vi "Check All Hardware Status.vi"(8 "error in (no error)":errorcluster caption="entrée d'erreur (pas d'erreur)", 11 "Control en entrée":refnum<class "Control-Server.lvclass">) -> (0 "error out":errorcluster caption="sortie d'erreur", 2 "HARDWARE":bool, 3 "Control en sortie":refnum<class "Control-Server.lvclass">)   [LabVIEW 2015, in "Control-Server.lvclass"]
uses:
  Control-Server.lvclass
  dependecies/ControlsVIs/Clusters-def/Message types.ctl
  dependecies/ControlsVIs/Clusters-def/Standard Command.ctl
  dependecies/ControlsVIs/Clusters-def/SERVER-Commands.ctl
  dependecies/ControlsVIs/Clusters-def/CONTROL-Reply-Allconnect.ctl
  Control-Server.lvclass/Control-Server.ctl
  GeneralFunctionality/GeneralFunctionality.lvclass/GeneralFunctionality.ctl
  Delay Line/DelayLine.lvclass
  Detector/Detector.lvclass
  Oscilloscope/Oscilloscope.lvclass
  DAQmxTasks/DAQmxTaskContainer/DAQmxTaskContainer.lvclass
  Message/Message.lvclass
  GeneralFunctionality/GeneralFunctionality.lvclass
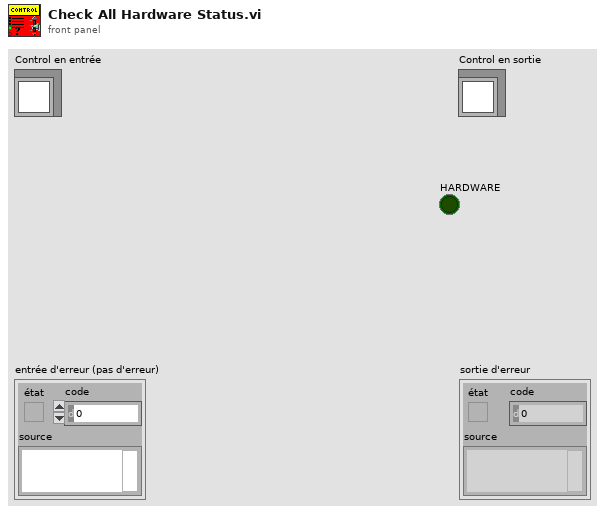
[diagram p1: front panel]
types:
  T1 = typedef "Control-Server.lvclass/CONTROL-Reply-Allconnect.ctl" = cluster{"On/Off":bool, "error":errorcluster}
  T2 = typedef "Control-Server.lvclass/SERVER-Commands.ctl" = string
  T3 = typedef "Standard Command.ctl" = cluster{"command":string, "data":variant}
  T4 = typedef "Message types.ctl" = string
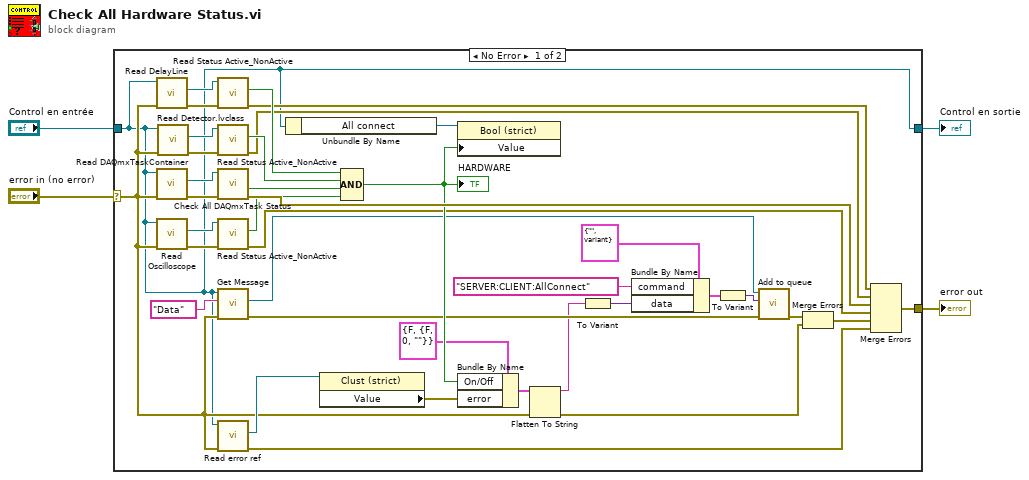
[diagram p0: block diagram]
diagram:
  n1 = case shown="No Error" "error in (no error)" {
    selector: "error in (no error)" -> [w13 w44]
    tunnel: [w30 w44] -> w3
    tunnel: [w6 w43] -> w1
    tunnel: "Control en entrée" -> [w6 w43]
    frame No Error {
      n2 = call "Read DelayLine.vi"("error in (no error)"=w13, "Control in"=w6) -> ("error out"=w40:errorcluster, "DelayLine.lvclass"=w39:refnum<class "DelayLine.lvclass">)  [unwired: 7 in, 1 out]
      n3 = call-dynamic "Read DAQmxTaskContainer.vi"("error in (no error)"=w13, "Control in"=w6) -> ("error out"=w38:errorcluster, "DAQmxTaskContainer.lvclass"=w37:refnum<class "DAQmxTaskContainer.lvclass">)  [unwired: 7 in, 1 out]
      n4 = call "Read Oscilloscope.vi"("error in (no error)"=w13, "Control-Server en entrée"=w6) -> ("error out"=w12:errorcluster, "Oscilloscope.lvclass"=w11:refnum<class "Oscilloscope.lvclass">)  [unwired: 7 in, 1 out]
      n5 = call "Read Detector.lvclass.vi"("error in (no error)"=w13, "Control in"=w6) -> ("error out"=w42:errorcluster, "Detector.lvclass"=w41:refnum<class "Detector.lvclass">)  [unwired: 7 in, 1 out]
      n6 = call "Read Status Active_NonActive.vi"("error in (no error)"=w40, "GeneralFunctionality in"=w39) -> ("error out"=w33:errorcluster, "Status Active/NonActive"=w36:bool)  [unwired: 7 in, 1 out]
      n7 = call "Read Status Active_NonActive.vi"("error in (no error)"=w42, "GeneralFunctionality in"=w41) -> ("error out"=w32:errorcluster, "Status Active/NonActive"=w35:bool)  [unwired: 7 in, 1 out]
      n8 = call "Check All DAQmxTask Status.vi"("error in (no error)"=w38, "DAQmxTaskContainer en entrée"=w37) -> ("error out"=w31:errorcluster, "One at least active"=w34:bool)  [unwired: 6 in, 2 out]
      n9 = call "Read Status Active_NonActive.vi"("error in (no error)"=w12, "GeneralFunctionality in"=w11) -> ("error out"=w9:errorcluster, "Status Active/NonActive"=w10:bool)  [unwired: 7 in, 1 out]
      n10 = call "Get Message.vi"("error in (no error)"=w13, "Message type"=T4 "Data", "GeneralFunctionality en entrée"=w6) -> ("error out"=w28:errorcluster, "Message.lvclass"=w26:refnum<class "Message.lvclass">)  [unwired: 6 in, 1 out]
      n11 = call "Read error ref.vi"("error in (no error)"=w13, "GeneralFunctionality in"=w6) -> ("error out"=w7:errorcluster, "error"=w17:refnum<vi>)  [unwired: 7 in, 1 out]
      n12 = Unbundle By Name(w6) -> ("All connect"=w5:refnum<vi>)
      n13 = property class="Clust (strict)"(reference=w17) -> ("Value"=w19:errorcluster)  [unwired: 1 in, 2 out]
      n14 = Compound Arithmetic op=AND ("Opérateur arithmétique")(w36, w35, w34, w10) -> (w29:bool)
      "HARDWARE" <- w29
      n15 = property class="Bool (strict)"(reference=w5, "Value"=w29) -> ()  [unwired: 1 in, 2 out]
      n16 = Bundle By Name(cluster=T1 {"On/Off"=FALSE, "error"={"status"=FALSE, "code"=0, "source"=""}} ("output cluster"), "On/Off"=w29, "error"=w19) -> (w16:T1)
      n17 = Flatten To String(anything=w16, error in (no error)=w13) -> (data string=w15:string, error out=w14:errorcluster)  [unwired: 2 in, 1 out]
      n18 = To Variant(anything=w15) -> (Variant=w22:variant)
      n19 = Bundle By Name(cluster=T3 {"command"="", "data"=variant} ("input cluster"), "command"=T2 "SERVER:CLIENT:AllConnect" ("Commands"), "data"=w22) -> (w21:T3)
      n20 = To Variant(anything=w21) -> (Variant=w20:variant)
      n21 = call "Add to queue.vi"("error in (no error)"=w28, "Data"=w20, "Message in"=w26) -> ("error out"=w18:errorcluster)  [unwired: 7 in, 1 out]
      n22 = Merge Errors(w18, w14) -> (w8:errorcluster)
      n23 = Merge Errors(w33, w32, w31, w9, w8, w7) -> (w30:errorcluster)
    }
    frame Error {
    }
  }
  "error out" <- w3
  "Control en sortie" <- w1
